vi "Alignment.vi"(0 "Sensor":enum16{"Ultrasonic", "Camera", "Gyro"}(ring)) -> ()   [LabVIEW 2013]
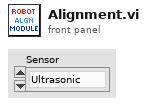
[diagram p1: front panel]
types:
  T1 = typedef "TargetType.ctl" = enum16{"Not Hot", "Hot"}
  T2 = cluster{"Scores":cluster{"Total":dbl, "Left":dbl, "Right":dbl, "Ratio":dbl, "Vertical":dbl, "index":i32, "State":T1}, "Verticals":cluster{"Horizontal?":bool, "Aspect Score":dbl, "Rect Score":dbl, cluster{"Left":dbl, "Top":dbl, "Right":dbl, "Bottom":dbl}, "Equiv H":dbl, "Equiv V":dbl}, "Horizontals":cluster{"Horizontal?":bool, "Aspect Score":dbl, "Rect Score":dbl, cluster{"Left":dbl, "Top":dbl, "Right":dbl, "Bottom":dbl}, "Equiv H":dbl, "Equiv V":dbl}, "Distance ft":dbl, "Center":cluster{"X":dbl, "Y":dbl}}[]
  T3 = cluster{"Scores":cluster{"Total":dbl, "Left":dbl, "Right":dbl, "Ratio":dbl, "Vertical":dbl, "index":i32, "State":T1}, "Verticals":cluster{"Horizontal?":bool, "Aspect Score":dbl, "Rect Score":dbl, cluster{"Left":dbl, "Top":dbl, "Right":dbl, "Bottom":dbl}, "Equiv H":dbl, "Equiv V":dbl}, "Horizontals":cluster{"Horizontal?":bool, "Aspect Score":dbl, "Rect Score":dbl, cluster{"Left":dbl, "Top":dbl, "Right":dbl, "Bottom":dbl}, "Equiv H":dbl, "Equiv V":dbl}, "Distance ft":dbl, "Center":cluster{"X":dbl, "Y":dbl}}
  T4 = cluster{"Horizontal?":bool, "Aspect Score":dbl, "Rect Score":dbl, cluster{"Left":dbl, "Top":dbl, "Right":dbl, "Bottom":dbl}, "Equiv H":dbl, "Equiv V":dbl}
  T5 = cluster{"Left":dbl, "Top":dbl, "Right":dbl, "Bottom":dbl}
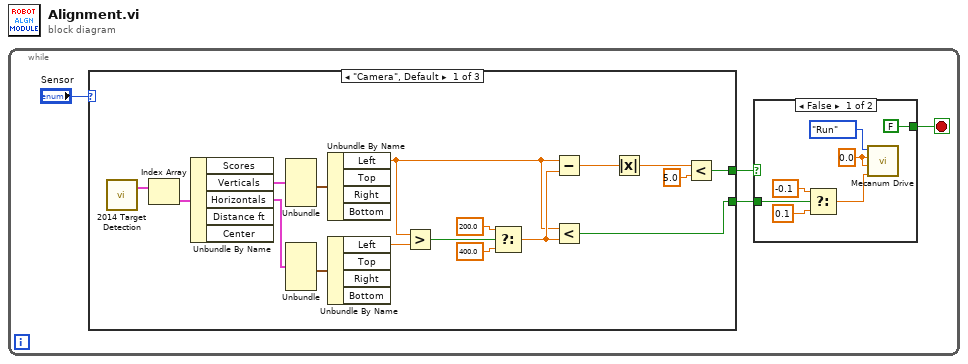
[diagram p0: block diagram]
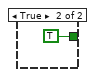
[diagram p2: hidden frame]
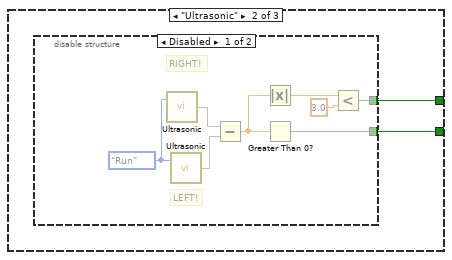
[diagram p3: hidden frame]
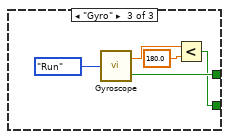
[diagram p5: hidden frame]
diagram:
  n1 = while {
    stop <- w2 stop-if-true
    n2 = case shown="\"Camera\", Default" "Sensor" {
      tunnel: [w13 w30 w40] -> w3
      tunnel: [w14 w31 w41] -> w4
      frame "Camera", Default {
        n3 = call "2014 Target Detection.vi"() -> ("Target Info"=w23:T2)  [unwired: 1 in, 1 out]
        n4 = Index Array(array=w23) -> (element=w22:T3)  [unwired: 1 in]
        n5 = Unbundle By Name(w22) -> ("Verticals"=w21:T4, "Horizontals"=w20:T4)  [unwired: 3 out]
        n6 = Unbundle(w21) -> (w19:T5)  [unwired: 5 out]
        n7 = Unbundle(w20) -> (w18:T5)  [unwired: 5 out]
        n8 = Unbundle By Name(w19) -> ("Left"=w15:dbl)  [unwired: 3 out]
        n9 = Unbundle By Name(w18) -> ("Left"=w17:dbl)  [unwired: 3 out]
        n10 = Greater?(x=w15, y=w17) -> (0:w26:bool)
        n11 = Select(t=200.0 ("y"), s=w26, f=400.0 ("y")) -> (s? t:f=w16:dbl)
        n12 = Subtract(x=w15, y=w16) -> (x-y=w29:dbl)
        n13 = Less?(x=w15, y=w16) -> (x < y?=w13:bool)
        n14 = Absolute Value(x=w29) -> (abs(x)=w28:dbl)
        n15 = Less?(x=w28, y=5.0) -> (x < y?=w14:bool)
      }
      frame "Ultrasonic" {
        n16 = disable-structure shown="Disabled" {
          disable-tunnel: [w35 _] -> w31
          disable-tunnel: [w33 _] -> w30
          frame Disabled {
            w32 = enum16{"Open", "Run", "End"}."Run" ("State Control")
            # "LEFT!"
            # "RIGHT!"
            n17 = call "Ultrasonic.vi"("State Control"=w32) -> (0:w37)  [unwired: 1 in]
            n18 = call "Ultrasonic.vi"("State Control"=w32) -> (0:w36)  [unwired: 1 in]
            n19 = Subtract(x=w37, y=w36) -> (x-y=w34:dbl)
            n20 = Absolute Value(x=w34) -> (abs(x)=w39:dbl)
            n21 = Greater Than 0?(x=w34) -> (x > 0?=w33:bool)
            n22 = Less?(x=w39, y=3.0) -> (x < y?=w35:bool)
          }
          frame Enabled {
          }
        }
      }
      frame "Gyro" {
        n23 = call "Gyroscope.vi"("State Control"=enum16{"Open", "Run", "End"}."Run") -> ("Angle"=w42:dbl, "Initial Position?"=w41:bool)
        n24 = Less?(x=w42, y=180.0) -> (x < y?=w40:bool)
      }
    }
    n25 = case shown="False" w4 {
      tunnel: [FALSE TRUE] -> w2
      tunnel: w3 -> [w8 _]
      frame False {
        w5 = 0.0 ("Strafing")
        n26 = Select(t=-0.1 ("Turning"), s=w8, f=0.1 ("Turning")) -> (s? t:f=w6:dbl)
        n27 = call "Mecanum Drive.vi"("Turn"=w6, "Forward/Backward"=w5, "Strafe"=w5, "State Control"=enum16{"Open", "Run", "End"}."Run") -> ()  [unwired: 4 in]
      }
      frame True {
      }
    }
  }
